vi "颜色模板.vi"(1 "Color":T1(ring)) -> (0 "ColorModule":cluster{u32, u32}[](array[cluster]))   [LabVIEW 2015]
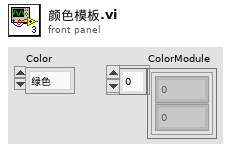
[diagram p1: front panel]
types:
  T1 = enum16{"绿色", "黄色", "蓝色", "紫色", "红色", "棕色", "橙色", "白色"}
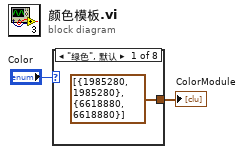
[diagram p0: block diagram]
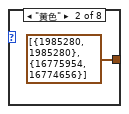
[diagram p2: hidden frame]
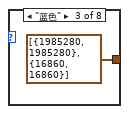
[diagram p3: hidden frame]
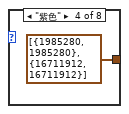
[diagram p4: hidden frame]
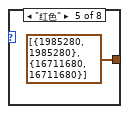
[diagram p5: hidden frame]
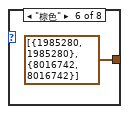
[diagram p6: hidden frame]
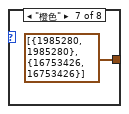
[diagram p7: hidden frame]
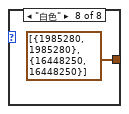
[diagram p8: hidden frame]
diagram:
  n1 = case shown="\"绿色\", 默认" "Color" {
    tunnel: [cluster{u32, u32}[] [{1985280, 1985280}, {6618880, 6618880}] cluster{u32, u32}[] [{1985280, 1985280}, {16775954, 16774656}] cluster{u32, u32}[] [{1985280, 1985280}, {16860, 16860}] cluster{u32, u32}[] [{1985280, 1985280}, {16711912, 16711912}] cluster{u32, u32}[] [{1985280, 1985280}, {16711680, 16711680}] cluster{u32, u32}[] [{1985280, 1985280}, {8016742, 8016742}] cluster{u32, u32}[] [{1985280, 1985280}, {16753426, 16753426}] cluster{u32, u32}[] [{1985280, 1985280}, {16448250, 16448250}]] -> w2
    frame "绿色", Default {
    }
    frame "黄色" {
    }
    frame "蓝色" {
    }
    frame "紫色" {
    }
    frame "红色" {
    }
    frame "棕色" {
    }
    frame "橙色" {
    }
    frame "白色" {
    }
  }
  "ColorModule" <- w2
